vi "Adjust Splitter.vi"(8 "error in":errorcluster, 9 "Show":bool, 10 "Splitter Info":T1, 11 "Bottom in":refnum<class "Bottom.lvclass">) -> (0 "error out":errorcluster, 3 "Bottom out":refnum<class "Bottom.lvclass">)   [LabVIEW 2023, in "Bottom.lvlib" / "Bottom.lvclass"]
doc: "The Adjust Splitter overrides the <b>Engine</b> Adjust Splitter routine.\n\nUsing the boundary definitions of the bottom panel actor, and the pointer to the splitter, this routine commands the splitter to:\n\n<b>Show = TRUE</b> Move the splitter up from the bottom of the screen\n <b>Show = FALSE</b> Return the splitter to the bottom of the screen"
uses:
  Project/Bottom.lvclass
  builds/Engine/Engine.lvlibp/Accessors/Read VI_Ref.vi
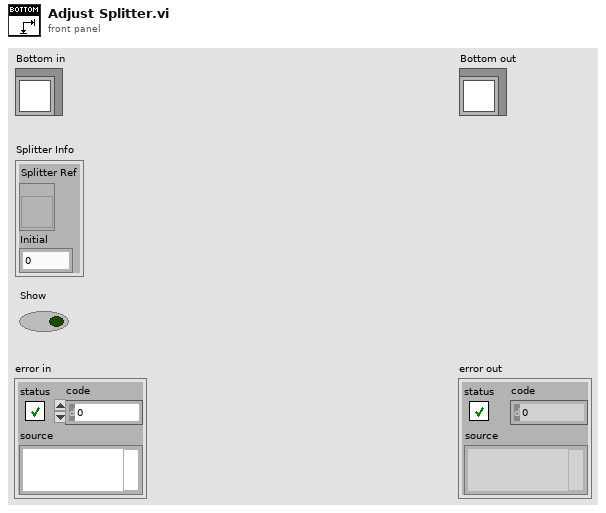
[diagram p1: front panel]
types:
  T1 = cluster{"Splitter Ref":refnum<vi>, "Initial":i32}
  T2 = typedef "LVPointTypeDef.ctl" = cluster{"Horizontal":i16, "Vertical":i16}
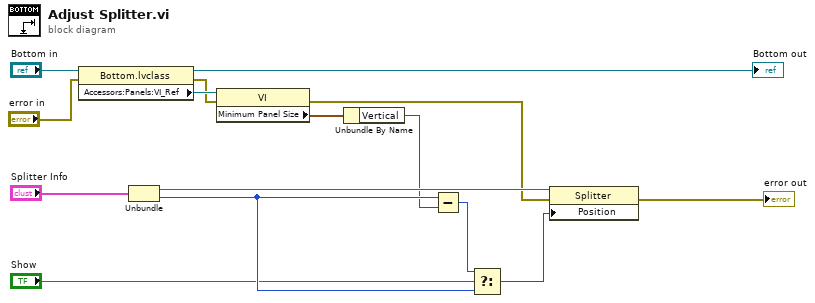
[diagram p0: block diagram]
diagram:
  n1 = property class="Bottom.lvclass"(reference="Bottom in", error in="error in") -> (reference out=→"Bottom out":refnum<class "Bottom.lvclass">, error out=w4:errorcluster, "Accessors:Panels:VI_Ref"=w14:refnum<vi>)
  n2 = Unbundle("Splitter Info") -> ("Splitter Ref"=w11:refnum<vi>, "Initial"=w9:i32)
  n3 = property class="VI"(reference=w14, error in=w4) -> (error out=w2:errorcluster, "Minimum Panel Size"=w13:T2)  [unwired: 1 out]
  n4 = Unbundle By Name(w13) -> ("Vertical"=w8:i16)
  n5 = Subtract(x=w9, y=w8) -> (x-y=w7:i32)
  n6 = Select(t=w7, s="Show", f=w9) -> (s? t:f=w10:i32)
  n7 = property class="Splitter"(reference=w11, error in=w2, "Position"=w10) -> (error out=→"error out":errorcluster)  [unwired: 1 out]
